vi "Create_distributed_array.vi"(0 "Upper Lim":dbl, 1 "Lower Lim":dbl, 2 "Num Points":i32, 4 "Distribution (lin)":enum16{"linear", "logarithmic"}(ring)) -> (5 "Array":dbl[](array[numeric]))   [LabVIEW 2016, in "Nanonis Prog Interface.lvlib"]
uses:
  Nanonis Prog Interface.lvlib
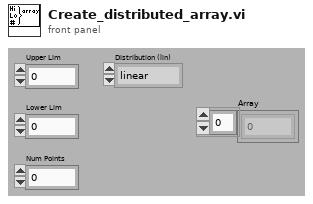
[diagram p1: front panel]
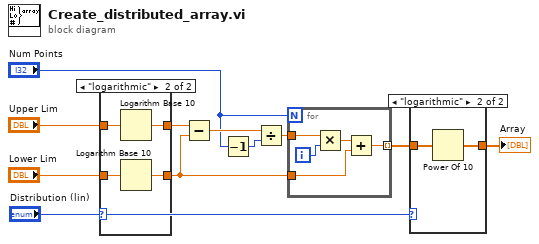
[diagram p0: block diagram]
diagram:
  n1 = case shown="\"logarithmic\"" "Distribution (lin)" {
    tunnel: "Upper Lim" -> [w13 w17]
    tunnel: [w13 w16] -> w6
    tunnel: "Lower Lim" -> [w12 w15]
    tunnel: [w12 w14] -> w4
    frame "linear" {
    }
    frame "logarithmic" {
      n2 = Logarithm Base 10(1:w17) -> (0:w16:dbl)
      n3 = Logarithm Base 10(1:w15) -> (0:w14:dbl)
    }
  }
  n4 = Subtract(x=w6, y=w4) -> (x-y=w11:dbl)
  n5 = Decrement(x="Num Points") -> (x-1=w8:i32)
  n6 = Divide(x=w11, y=w8) -> (x/y=w10:dbl)
  n7 = for {
    N: "Num Points" -> [_]
    tunnel: w10 -> [w22]
    tunnel: w4 -> [w19]
    tunnel: [w18] -> w2 mode=indexing
    i -> [w21]
    n8 = Multiply(x=w22, y=w21) -> (x*y=w20:dbl)
    n9 = Add(x=w20, y=w19) -> (x+y=w18:dbl)
  }
  n10 = case shown="\"logarithmic\"" "Distribution (lin)" {
    tunnel: w2 -> [w23 w25]
    tunnel: [w23 w24] -> w1
    frame "linear" {
    }
    frame "logarithmic" {
      n11 = Power Of 10(x=w25) -> (10^x=w24:dbl[])
    }
  }
  "Array" <- w1
